vi "Analyze coinc array after hunt.vi"(11 "Array":T1(array[cluster])) -> (2 "Largest array size":i32, 3 "All equal?":bool)   [LabVIEW 2016]
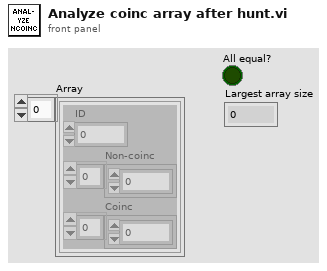
[diagram p1: front panel]
types:
  T1 = cluster{"ID":i8, "Non-coinc":u64[], "Coinc":u64[]}[]
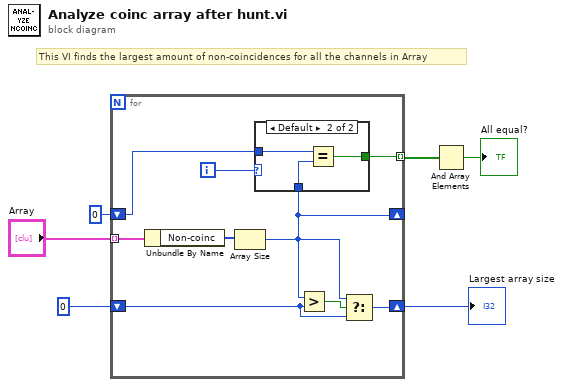
[diagram p0: block diagram]
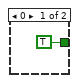
[diagram p2: hidden frame]
diagram:
  # "This VI finds the largest amount of non-coincidences for all the channels in Array"
  n1 = for {
    tunnel: "Array" -> [w15] mode=indexing
    shift-right: [w8] -> _
    shift-left: 0 -> [w13]
    tunnel: [w12] -> w5 mode=indexing
    shift-right: [w9] -> w1
    shift-left: 0 -> [w7]
    i -> [w11]
    n2 = Unbundle By Name(w15) -> ("Non-coinc"=w14:u64[])
    n3 = Array Size(array=w14) -> (size(s)=w8:i32)
    n4 = case shown="Default" w11 {
      tunnel: w13 -> [_ w19]
      tunnel: w8 -> [_ w18]
      tunnel: [TRUE w17] -> w12
      frame 0 {
      }
      frame Default {
        n5 = Equal?(x=w19, y=w18) -> (x = y?=w17:bool)
      }
    }
    n6 = Greater?(x=w8, y=w7) -> (0:w10:bool)
    n7 = Select(t=w8, s=w10, f=w7) -> (s? t:f=w9:i32)
  }
  "Largest array size" <- w1
  n8 = And Array Elements(Boolean array=w5) -> (logical AND=→"All equal?":bool)
